vi "Configure User-Defined Codes.vi"(8 "Error In":errorcluster, 11 "User-Defined Codes":i32[](array[numeric])) -> (0 "Error Out":errorcluster)   [LabVIEW 2014, in "Logger.lvlib"]
uses:
  Logger.lvlib
  Private/_Error Handler Configuration Action.ctl
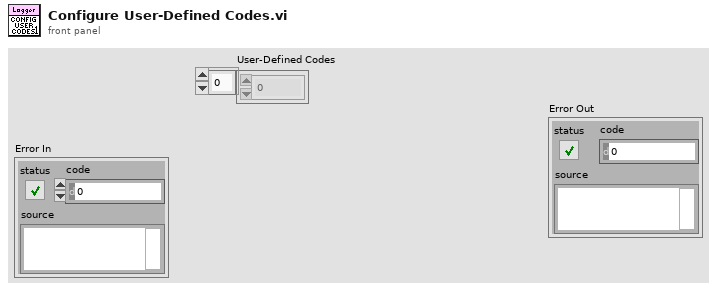
[diagram p1: front panel]
types:
  T1 = typedef "Logger.lvlib/_Error Handler Configuration Action.ctl" = enum16{"Initialize", "Get", "Set Verbosity", "Set User-Defined Codes", "Set User-Defined Descriptions", "Shutdown"}
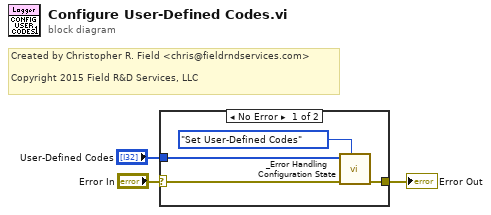
[diagram p0: block diagram]
diagram:
  # "Created by Christopher R. Field <chris@fieldrndservices.com>\n\nCopyright 2015 Field R&D Services, LLC"
  n1 = case shown="No Error" "Error In" {
    selector: "Error In" -> [w7 w8]
    tunnel: [w6 w8] -> w2
    tunnel: "User-Defined Codes" -> [w4 _]
    frame No Error {
      n2 = call "_Error Handling Configuration State.vi"("Action"=_Error_Handler_Configuration_Action."Set User-Defined Codes", "Error In"=w7, "Set Value"=w4) -> ("Error Out"=w6:errorcluster)  [unwired: 7 in, 1 out]
    }
    frame Error {
    }
  }
  "Error Out" <- w2
